vi "Icon Editor.vi"(8 "error in (no error)":errorcluster, 10 "Glyph":string(combo), 11 "Glyph Source in":refnum<class "Glyph Source.lvclass">) -> (0 "error out":errorcluster, 3 "Glyph Source out":refnum<class "Glyph Source.lvclass">)   [LabVIEW 2023, in "LV-Awesome.lvlib"]
uses:
  LV-Awesome.lvlib
  Font Glyph Drawer Interface/Picture Control Canvas/Picture Control Canvas.lvclass
  Font Glyph Drawer Interface/Glyph Canvas/Glyph Canvas.lvclass
  Font Glyph Drawer Interface/Glyph Source/Glyph Source.lvclass
  LV Awesome/LV Awesome.lvclass
  Font Glyph Drawer Interface/Static Image Transform/Static Image Transform.lvclass
  Freetype Drawer/Freetype Drawer/Freetype Drawer.lvclass
panel:
  in  "Alpha":u8(slide)=255 scale=0.0..255.0
  in  "Back":u32(colorbox)=16448250
  in  "Front":u32(colorbox)
  in  "Transform":T1={"Offset"={"Left"=0.0, "Top"=0.0}, "Scale"={"Width"=100.0, "Height"=100.0}, "Rotate"=0.0, "Translate"={"Left"=0.0, "Top"=0.0}, "Origin at Center"=TRUE, "Center on Canvas"=TRUE} {"Rotate" scale=0.0..360.0; "Scale"."Height" format="%#_g %"; "Scale"."Width" format="%#_g %"}
  in  "Copy":bool
  in  "Font Size":dbl(slide)=64.0 scale=0.0..100.0
  in  "Exit":bool
  in  "Symbol Size":cluster{"Width":u16, "Height":u16}={"Width"=128, "Height"=128}
  out "Symbol":picture
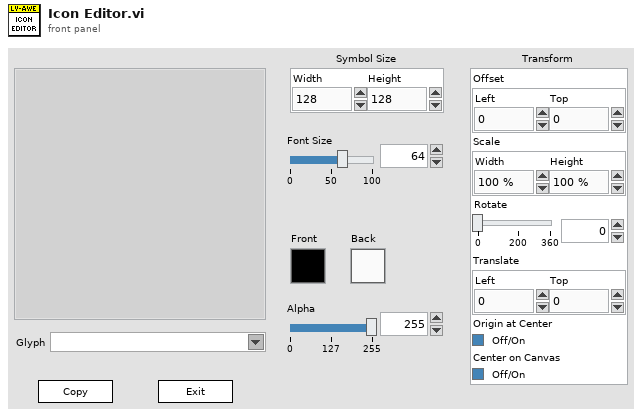
[diagram p1: front panel]
types:
  T1 = cluster{"Offset":cluster{"Left":dbl, "Top":dbl}, "Scale":cluster{"Width":dbl, "Height":dbl}, "Rotate":dbl, "Translate":cluster{"Left":dbl, "Top":dbl}, "Origin at Center":bool, "Center on Canvas":bool}
  T2 = cluster{"Front":cluster{"Color":u32, "Alpha":u8}, "Back":cluster{"Color":u32, "Alpha":u8}}
  T3 = typedef "imagedata.ctl" = cluster{"image type":i32, "image depth":i32, "image":u8[], "mask":u8[], "colors":u32[], "Rectangle":cluster{"left":i16, "top":i16, "right":i16, "bottom":i16}}
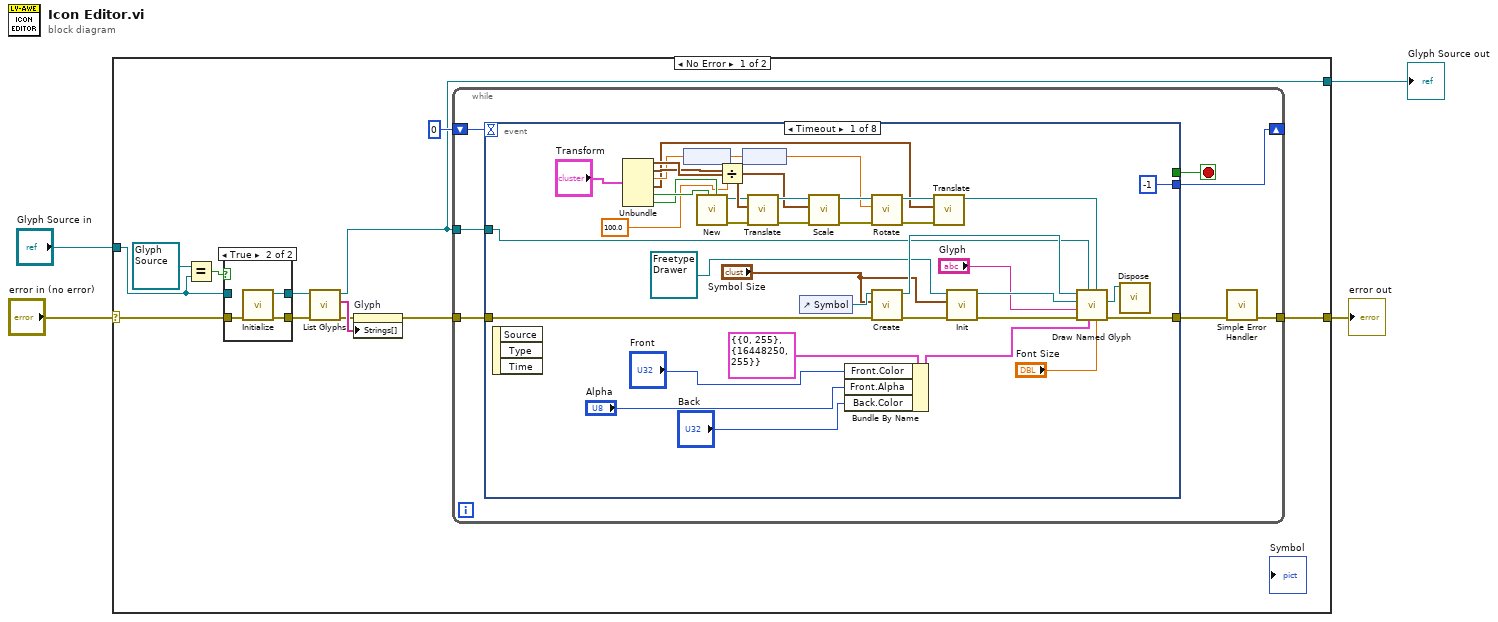
[diagram p0: block diagram]
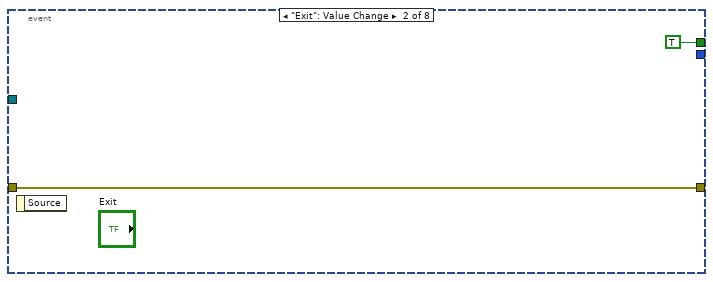
[diagram p3: hidden frame]
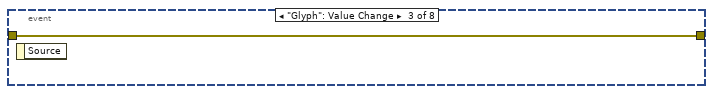
[diagram p4: hidden frame]
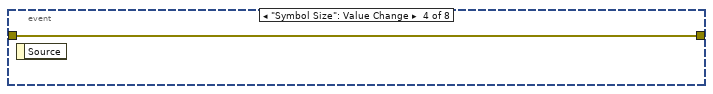
[diagram p5: hidden frame]
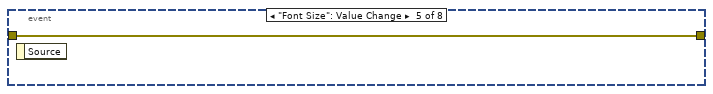
[diagram p6: hidden frame]
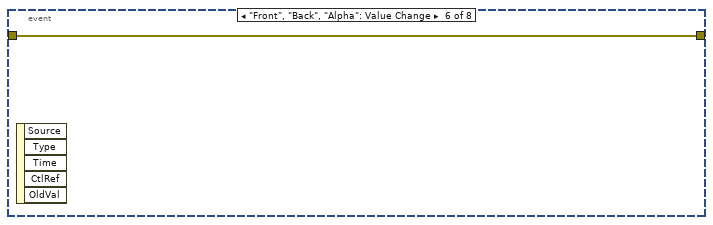
[diagram p7: hidden frame]
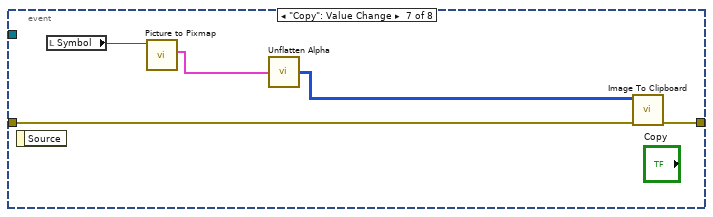
[diagram p8: hidden frame]
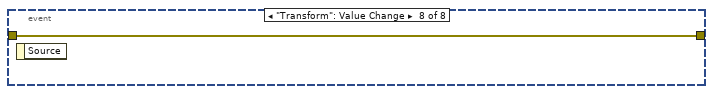
[diagram p9: hidden frame]
diagram:
  n1 = case shown="No Error" "error in (no error)" {
    selector: "error in (no error)" -> [w9 w81]
    tunnel: [w12 w81] -> w3
    tunnel: [w11 w80] -> w2
    tunnel: "Glyph Source in" -> [w5 w80]
    frame No Error {
      n2 = Equal?(x=refnum<class "Glyph Source.lvclass"> refnum, y=w5) -> (x = y?=w7:bool)
      n3 = case shown="True" w7 {
        tunnel: w9 -> [w18 w21]
        tunnel: [w18 w20] -> w8
        tunnel: [w17 w19] -> w6
        tunnel: w5 -> [w17 _]
        frame False {
        }
        frame True {
          n4 = call "Initialize.vi"("error out 2"=w21) -> ("error out"=w20:errorcluster, "LV Awesome"=w19:refnum<class "LV Awesome.lvclass">)  [unwired: 9 in]
        }
      }
      n5 = call-dynamic "List Glyphs.vi"("error in (no error)"=w8, "Glyph Source in"=w6) -> ("error out"=w15:errorcluster, "Glyphs"=w16:string[], "Glyph Source out"=w11:refnum<class "Glyph Source.lvclass">)  [unwired: 7 in]
      n6 = property on="Glyph" class="CmbBox"(error in=w15, "Strings[]"=w16) -> (error out=w13:errorcluster)  [unwired: 1 in, 1 out]
      n7 = while {
        shift-right: [w27] -> _
        shift-left: 0 -> [w28]
        tunnel: w13 -> [w26]
        tunnel: [w22] -> w12
        tunnel: w11 -> [w24]
        stop <- w23 stop-if-true
        n8 = event shown="[0] Timeout" {
          selector: _ -> [_ _ _ _ _ _ _ _]
          dyn-events: _ -> [_ _ _ _ _ _ _ _]
          timeout: w28 -> [_ _ _ _ _ _ _ _]
          tunnel: [-1 _ _ _ _ _ _ _] -> w27
          tunnel: w26 -> [w65 w68 w70 w71 w72 w73 w77 w79]
          tunnel: [w64 w68 w70 w71 w72 w73 w76 w79] -> w25
          tunnel: w24 -> [w62 _ _ _ _ _ _ _]
          tunnel: [_ TRUE _ _ _ _ _ _] -> w23
          event Timeout {
            n9 = event-data() -> ()  [unwired: 1 in, 3 out]
            n10 = Unbundle("Transform") -> ("Offset"=w48:cluster{"Left":dbl, "Top":dbl}, "Scale"=w47:cluster{"Width":dbl, "Height":dbl}, "Rotate"=w46:dbl, "Translate"=w43:cluster{"Left":dbl, "Top":dbl}, "Origin at Center"=w37:bool, "Center on Canvas"=w36:bool)
            n11 = node(w46) -> (w45:dbl[unit])
            n12 = call "New.vi"("Center on Canvas"=w36, "Origin at Center"=w37) -> ("error out"=w38:errorcluster, "Static Image Transform out"=w39:refnum<class "Static Image Transform.lvclass">)  [unwired: 8 in]
            n13 = Divide(x=w47, y=100.0) -> (x/y=w31:cluster{"Width":dbl, "Height":dbl})
            n14 = node(w45) -> (w44:dbl)
            n15 = call "Translate.vi"("error in (no error)"=w38, "Translation"=w48, "Static Image Transform in"=w39) -> ("error out"=w40:errorcluster, "Static Image Transform out"=w53:refnum<class "Static Image Transform.lvclass">)  [unwired: 7 in]
            n16 = control-ref of="Symbol"() -> (w67:refnum<vi>)
            n17 = call "Scale.vi"("error in (no error)"=w40, "Scale"=w31, "Static Image Transform in"=w53) -> ("error out"=w41:errorcluster, "Static Image Transform out"=w52:refnum<class "Static Image Transform.lvclass">)  [unwired: 7 in]
            n18 = Bundle By Name(cluster=T2 {"Front"={"Color"=0, "Alpha"=255}, "Back"={"Color"=16448250, "Alpha"=255}} ("Colors"), "Front.Color"="Front", "Front.Alpha"="Alpha", "Back.Color"="Back") -> (w35:T2)
            n19 = call "Rotate.vi"("error in (no error)"=w41, "Rotation rad"=w44, "Static Image Transform in"=w52) -> ("error out"=w42:errorcluster, "Static Image Transform out"=w51:refnum<class "Static Image Transform.lvclass">)  [unwired: 7 in]
            n20 = call "Create.vi"("error in (no error)"=w65, "Size (Full)"="Symbol Size", "2D Picture"=w67) -> ("error out"=w61:errorcluster, "Picture Control Canvas out"=w63:refnum<class "Picture Control Canvas.lvclass">)  [unwired: 7 in]
            n21 = call "Translate.vi"("error in (no error)"=w42, "Translation"=w43, "Static Image Transform in"=w51) -> ("Static Image Transform out"=w50:refnum<class "Static Image Transform.lvclass">)  [unwired: 7 in, 1 out]
            n22 = call-dynamic "Init.vi"("error in (no error)"=w61, "Size"="Symbol Size", "Class 1 in"=refnum<class "Freetype Drawer.lvclass"> refnum ("Freetype Drawer.lvlib:Freetype Drawer.lvclass")) -> ("error out"=w60:errorcluster, "Class 1 out"=w58:refnum<class "Freetype Drawer.lvclass">)  [unwired: 7 in]
            n23 = call "Draw Named Glyph.vi"("Size"="Font Size", "Transform (Center)"=w50, "Colors"=w35, "Glyph Source in"=w62, "error in (no error)"=w60, "Glyph Name"="Glyph", "Glyph Drawer in"=w58, "Glyph Canvas in"=w63) -> ("error out"=w64:errorcluster, "Glyph Drawer out"=w55:refnum<class "Freetype Drawer.lvclass">)  [unwired: 1 in, 1 out]
            n24 = call-dynamic "Dispose.vi"("Class 1 in"=w55) -> ()  [unwired: 10 in, 1 out]
          }
          event "Exit": Value Change {
            n25 = event-data() -> ()  [unwired: 1 in, 1 out]
          }
          event "Glyph": Value Change {
            n26 = event-data() -> ()  [unwired: 1 in, 1 out]
          }
          event "Symbol Size": Value Change {
            n27 = event-data() -> ()  [unwired: 1 in, 1 out]
          }
          event "Font Size": Value Change {
            n28 = event-data() -> ()  [unwired: 1 in, 1 out]
          }
          event "Front", "Back", "Alpha": Value Change {
            n29 = event-data() -> ()  [unwired: 1 in, 5 out]
          }
          event "Copy": Value Change {
            n30 = event-data() -> ()  [unwired: 1 in, 1 out]
            n31 = local read "Symbol"() -> (w78:picture)
            n32 = call <vilib>:"Picture to Pixmap.vi"("picture"=w78) -> ("image data"=w75:T3)  [unwired: 9 in, 1 out]
            n33 = call "Unflatten Alpha.vi"("image data"=w75) -> ("32-bit pixmap"=w74:u32[][])
            n34 = call "Image To Clipboard.vi"("error in (no error)"=w77, "24-bit pixmap"=w74) -> ("error out"=w76:errorcluster)  [unwired: 9 in]
          }
          event "Transform": Value Change {
            n35 = event-data() -> ()  [unwired: 1 in, 1 out]
          }
        }
        n36 = call <vilib>:"Simple Error Handler.vi"("error in (no error)"=w25) -> ("error out"=w22:errorcluster)  [unwired: 4 in, 4 out]
      }
    }
    frame Error {
    }
  }
  "error out" <- w3
  "Glyph Source out" <- w2
